vi "Generate Error Code.vi"(11 "Errors.nimxl file path":path=path "E:/Dev/ni-central/src/rfmx/NR/RFmxNRErrorFile/source/mxlErrorFiles/errors.nimxl") -> (2 "min value":i32, 3 "max value":i32)   [LabVIEW 2023]
uses:
  46010a91-3e5b-45c8-ad92-bda641e1b7f9.vi
  <vilib>/Utility/file.llb/Read Delimited Spreadsheet (string).vi
panel:
  out "Waveform Graph":i32[](graph)
  out "Suggested New Error Code":i32
  in  "Error Range":cluster{"Start":i32, "End":i32}={"Start"=-684100, "End"=-684149}
  out "New Error Code in specified range":i32
  out "Used Error Codes":i32[](array[numeric])
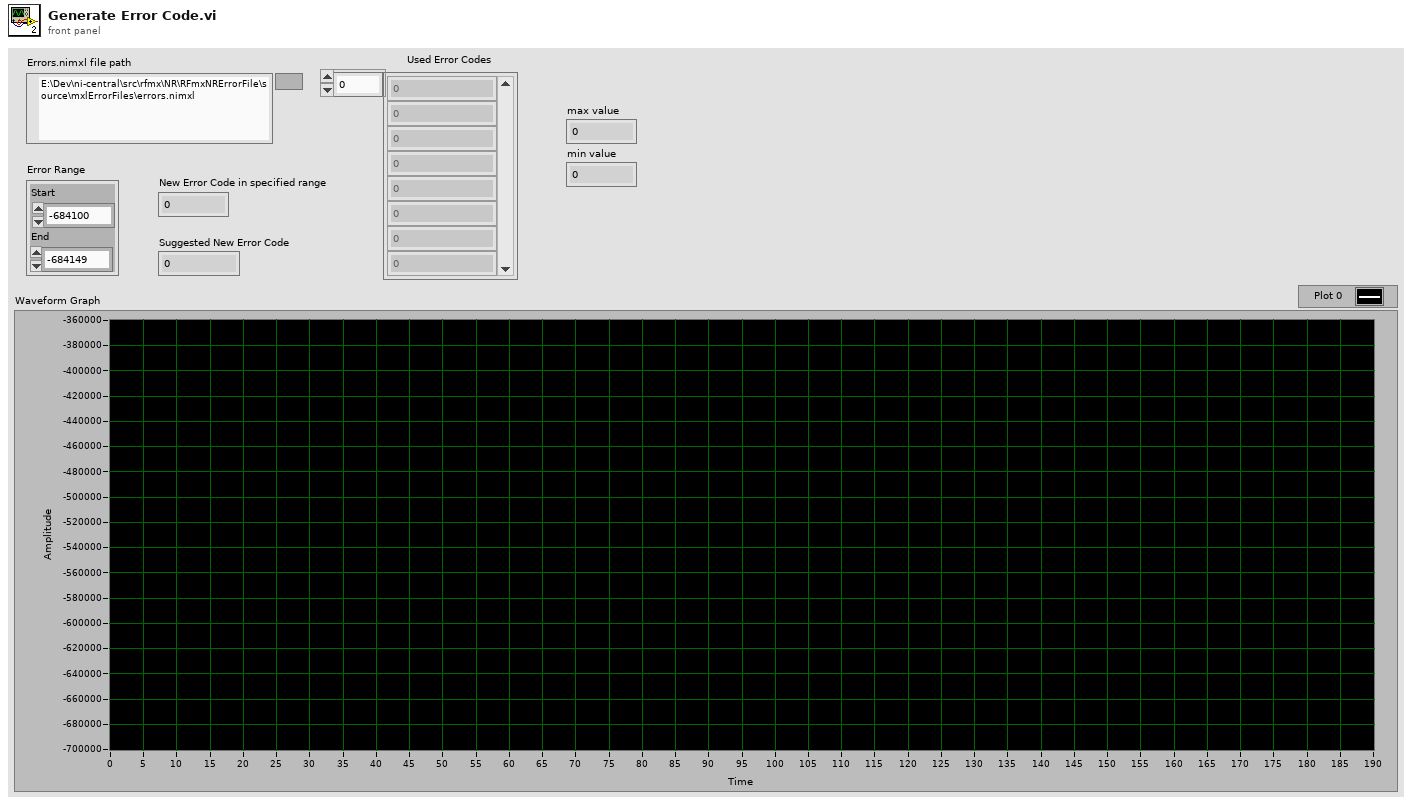
[diagram p1: front panel]
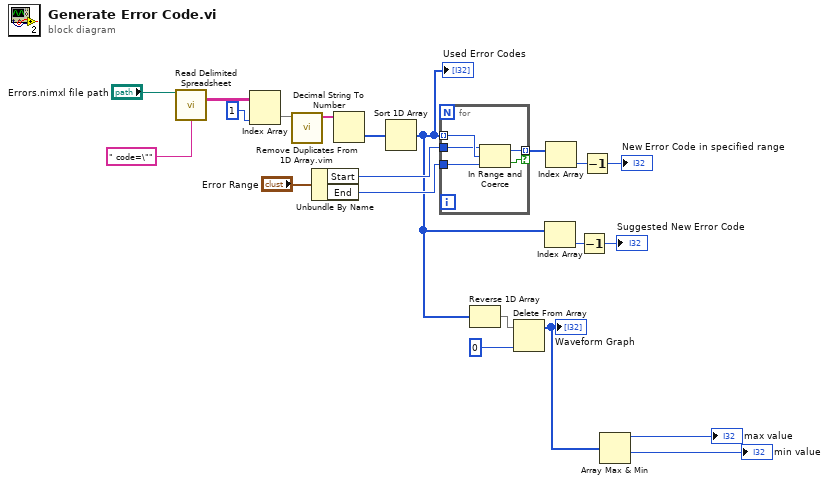
[diagram p0: block diagram]
diagram:
  n1 = call-poly <vilib>:"Read Delimited Spreadsheet.vi"("file path (dialog if empty)"="Errors.nimxl file path", "delimiter (\\t)"=" code=\"" ("delimiter (\\t)")) -> ("all rows"=w19:string[][])  [unwired: 8 in, 5 out]
  n2 = Index Array(array=w19, index (col)=1) -> (element=w17:string[])  [unwired: 1 in]
  n3 = call "Remove Duplicates From 1D Array.vim"("array"=w17) -> ("array with duplicates removed"=w16:string[])  [unwired: 10 in]
  n4 = Unbundle By Name("Error Range") -> ("Start"=w10:i32, "End"=w9:i32)
  n5 = Decimal String To Number(string=w16) -> (number=w15:i32[])  [unwired: 2 in, 1 out]
  n6 = Sort 1D Array(array=w15) -> (sorted array=w4:i32[])
  "Used Error Codes" <- w4
  n7 = for {
    tunnel: w4 -> [w26] mode=indexing
    tunnel: [w25] -> w12 mode=indexing if=w24
    tunnel: w10 -> [w23]
    tunnel: w9 -> [w22]
    n8 = In Range and Coerce(upper limit=w23, x=w26, lower limit=w22) -> (coerced(x)=w25:i32, In Range?=w24:bool)
  }
  n9 = Reverse 1D Array(array=w4) -> (reversed array=w6:i32[])
  n10 = Delete From Array(array=w6, index=0) -> (array with subset deleted=w3:i32[])  [unwired: 1 in, 1 out]
  "Waveform Graph" <- w3
  n11 = Index Array(array=w4) -> (element=w8:i32)  [unwired: 1 in]
  n12 = Index Array(array=w12) -> (element=w13:i32)  [unwired: 1 in]
  n13 = Decrement(x=w8) -> (x-1=→"Suggested New Error Code":i32)
  n14 = Decrement(x=w13) -> (x-1=→"New Error Code in specified range":i32)
  n15 = Array Max & Min(array=w3) -> (max value=→"max value":i32, min value=→"min value":i32)  [unwired: 2 out]
